vi "send.vi"(8 "Error In":errorcluster, 9 "Severity Code (error)":T1=enum."error", 10 "Message Content":string, 11 "Message Tag":string) -> (0 "Error Out":errorcluster)   [LabVIEW 2012, in "CS++MessageLogger.lvlib"]
doc: "Send mesage to central message logger."
uses:
  CS++MessageLogger.lvlib
  Base/Severity.ctl
  <userlib>/syslog/_subVIs/TypeDefs/syslog_facility_codes.ctl
  Base/CS++Base.lvlib
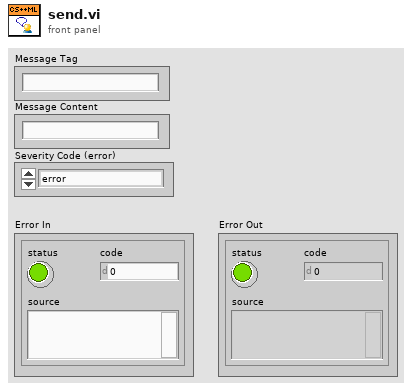
[diagram p1: front panel]
types:
  T1 = typedef "CS++Base.lvlib/Severity.ctl" = enum16{"emergency", "alert", "critical", "error", "warning", "notice", "info", "debug"}
  T2 = typedef "syslog_facility_codes.ctl" = enum16{"kernel", "user", "mail", "system daemons", "security/authorization", "syslogd", "line printer", "network news", "uucp", "clock daemon", "security/authorization (alternate)", "FTP daemon", "NTP subsystem", "log audit", "log alert", "clock daemon (alternate)", "local use 0", "local use 1", "local use 2", "local use 3", "local use 4", "local use 5", "local use 6", "local use 7"}
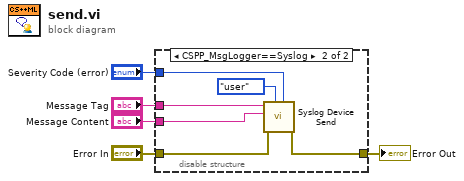
[diagram p0: block diagram]
diagram:
  n1 = disable-structure shown="CSPP_MsgLogger==Syslog" {
    disable-tunnel: "Message Tag" -> [_ w12]
    disable-tunnel: "Message Content" -> [_ w11]
    disable-tunnel: "Severity Code (error)" -> [_ w9]
    disable-tunnel: "Error In" -> [w6 w8]
    disable-tunnel: [w6 w7] -> w1
    frame condition #0 {
    }
    frame condition #1 (active) {
      n2 = call <userlib>:"Syslog Device Send.vi"("Severity Code (error)"=w9, "Facility Code (user)"=syslog_facility_codes."user", "error in (no error)"=w8, "Message Content"=w11, "Message Tag"=w12) -> ("error out"=w7:errorcluster)  [unwired: 5 in, 1 out]
    }
  }
  "Error Out" <- w1
